vi "photonDist.vi"() -> ()   [LabVIEW 2023]
uses:
  <vilib>/Rock Robotics/WPI/ThirdParty/PhotonVisionLib/PhotonVisionLib.lvlib
  <vilib>/Rock Robotics/WPI/ThirdParty/JAS_Junk/TrajLib/Trajectory_Library.lvlib
panel:
  in  "Gyro Reading (Deg)":dbl
  out "DistanceToTarget (Meters)":dbl
  out "Yaw Offset (Degrees)":dbl
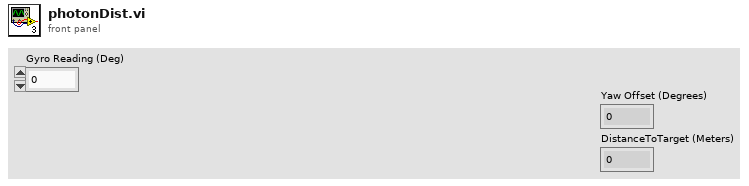
[diagram p1: front panel]
types:
  T1 = typedef "PhotonVisionLib.lvlib/PhotonPipelineResultType.ctl" = cluster{"TargetCount":i32, "Latency_MilliSec":dbl, "Targets":T2[], "TimeStampSec":dbl, "PhotonMultiTargetPNPResult":T8}
  T2 = typedef "PhotonVisionLib.lvlib/PhotonTrackedTargetType.ctl" = cluster{"Yaw":dbl, "Pitch":dbl, "Area":dbl, "Skew":dbl, "MinAreaRectCorners":T3[], "BestCameraToTarget":T4, "FiiducialId":i32, "AltCameraToTarget":T4, "PoseAmbiguity":dbl, "DetectedCorners":T3[]}
  T3 = typedef "PhotonVisionLib.lvlib/TargetCornerType.ctl" = cluster{"X":dbl, "Y":dbl}
  T4 = typedef "Trajectory_Library.lvlib/TRANSFORM3D.ctl" = cluster{"TRANSLATION3D":T5, "ROTATION3D":T6, "XF":bool}
  T5 = typedef "Trajectory_Library.lvlib/TRANSLATION3D.ctl" = cluster{"X":dbl, "Y":dbl, "Z":dbl}
  T6 = typedef "Trajectory_Library.lvlib/ROTATION3D.ctl" = cluster{"Q_quaternion":T7}
  T7 = typedef "Trajectory_Library.lvlib/QUATERNION.ctl" = cluster{"R":dbl, "V":dbl[]}
  T8 = typedef "PhotonVisionLib.lvlib/PhotonMultiTargetPNPResultType.ctl" = cluster{"PhotonPNPResult":T9, "FiducialIDsUsed":i16[]}
  T9 = typedef "PhotonVisionLib.lvlib/PhotonPNPResultType.ctl" = cluster{"IsPresent":bool, "bestReprojErr":dbl, "altReprojErr":dbl, "ambiguity":dbl, "Best":T4, "Alt":T4}
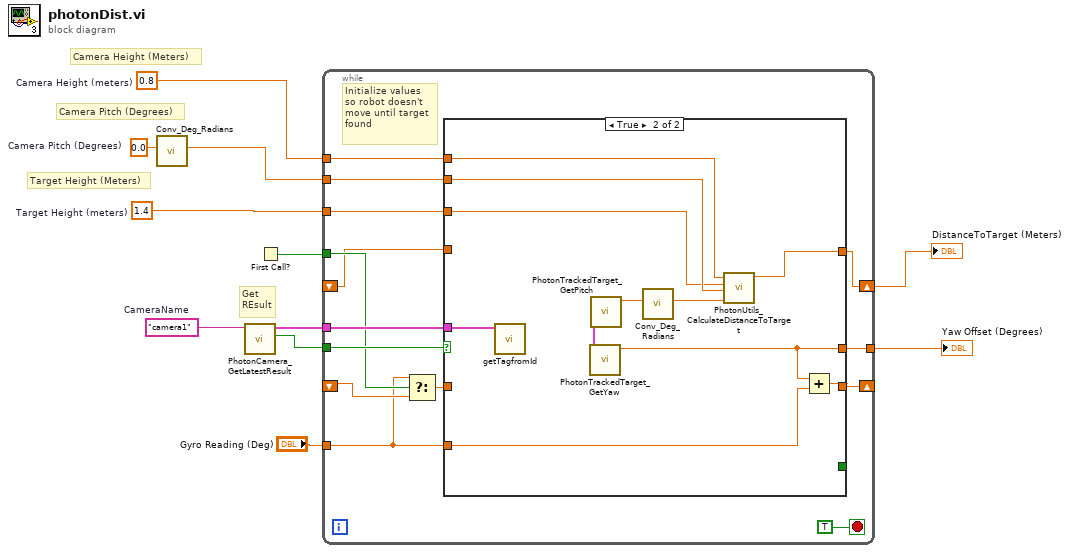
[diagram p0: block diagram]
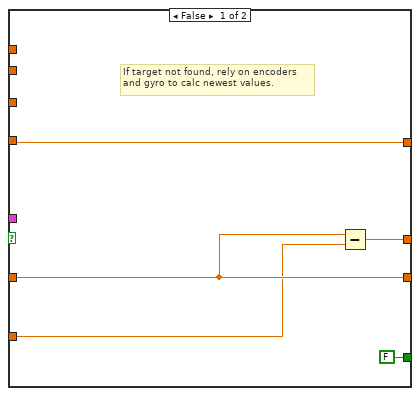
[diagram p2: hidden frame]
diagram:
  w7 = 1.4  # Target Height (meters)
  w5 = 0.8  # Camera Height (meters)
  w2 = 0.0  # Camera Pitch (Degrees)
  w1 = "camera1"  # CameraName
  # "Camera Pitch (Degrees)"
  # "Target Height (Meters)"
  # "Camera Height (Meters)"
  # "Get\nREsult"
  n1 = call <vilib>:"Conv_Deg_Radians.vi"("Degress"=w2) -> ("Radians"=w6:dbl)  [unwired: 10 in]
  n2 = call <vilib>:"PhotonCamera_GetLatestResult.vi"("CameraName"=w1) -> ("HasTargets"=w3:bool, "PipelineResult"=w4:T1)  [unwired: 7 in, 2 out]
  n3 = First Call?() -> (First Call?: T/F=w11:bool)
  n4 = while {
    tunnel: w3 -> [w25]
    tunnel: w4 -> [w24]
    tunnel: w5 -> [w23]
    tunnel: w6 -> [w22]
    tunnel: w7 -> [w21]
    tunnel: [w19] -> w9
    tunnel: "Gyro Reading (Deg)" -> [w13]
    shift-right: [w17] -> _
    shift-left: _ -> [w16]
    tunnel: w11 -> [w14]
    shift-right: [w20] -> w8
    shift-left: _ -> [w12]
    stop <- TRUE stop-if-true
    # "Initialize values\nso robot doesn't\nmove until target\nfound"
    n5 = Select(t=w13, s=w14, f=w16) -> (s? t:f=w15:dbl)
    n6 = case shown="True" w25 {
      tunnel: w24 -> [_ w31]
      tunnel: [w30 w34] -> w19
      tunnel: w23 -> [_ w38]
      tunnel: w22 -> [_ w37]
      tunnel: w21 -> [_ w36]
      tunnel: [w26 w35] -> w20
      tunnel: w13 -> [w28 w33]
      tunnel: [w29 w32] -> w17
      tunnel: w15 -> [w29 _]
      tunnel: [FALSE ("TargetFound") _] -> _
      tunnel: w12 -> [w26 _]
      frame False {
        # "If target not found, rely on encoders\nand gyro to calc newest values."
        n7 = Subtract(x=w29, y=w28) -> (x-y=w30:dbl)
      }
      frame True {
        n8 = call "getTagfromId.vi"("PipelineResult"=w31) -> ()  [unwired: 11 in]
        n9 = call <vilib>:"PhotonTrackedTarget_GetYaw.vi"() -> ("Yaw"=w34:dbl, "TrackedTarget"=w41:T2)  [unwired: 10 in]
        n10 = call <vilib>:"PhotonTrackedTarget_GetPitch.vi"("TrackedTarget"=w41) -> ("Pitch"=w40:dbl)  [unwired: 10 in]
        n11 = call <vilib>:"Conv_Deg_Radians.vi"("Degress"=w40) -> ("Radians"=w39:dbl)  [unwired: 10 in]
        n12 = call <vilib>:"PhotonUtils_CalculateDistanceToTarget.vi"("TargetPitch_Radians"=w39, "CameraPitch_Radians"=w37, "TargetHeight_Meters"=w36, "CameraHeight_Meters"=w38) -> ("DistanceToTarget_Meters"=w35:dbl)  [unwired: 7 in]
        n13 = Add(x=w34, y=w33) -> (x+y=w32:dbl)
      }
    }
  }
  "DistanceToTarget (Meters)" <- w8
  "Yaw Offset (Degrees)" <- w9
